vi "Channel.BuildDisplayedName.vi"(11 "String in":string) -> (3 "String out":string)   [LabVIEW 2013]
uses:
  NationalInstruments.VeriStand
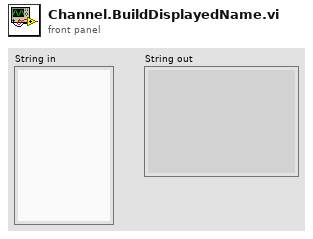
[diagram p1: front panel]
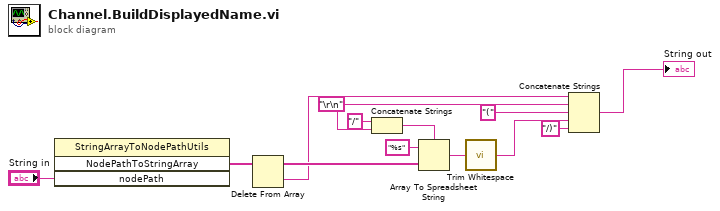
[diagram p0: block diagram]
diagram:
  w11 = "\r\n"
  n1 = invoke class="StringArrayToNodePathUtils" method="NodePathToStringArray"("nodePath"="String in") -> ("NodePathToStringArray"=w6:string[])  [unwired: 3 in, 3 out]
  n2 = Delete From Array(array=w6) -> (deleted portion=w7:string, array with subset deleted=w8:string[])  [unwired: 2 in]
  n3 = Concatenate Strings("/" ("string"), w11) -> (w10:string)
  n4 = Array To Spreadsheet String(delimiter (Tab)=w10, array=w8, 3:"%s" ("format string")) -> (spreadsheet string=w5:string)
  n5 = call <vilib>:"Trim Whitespace.vi"("string"=w5) -> ("trimmed string"=w3:string)  [unwired: 1 in]
  n6 = Concatenate Strings(w7, w11, "(" ("string"), w3, "/)" ("string")) -> (→"String out":string)
